vi "Select Level UI.vi"() -> (2 "Cancelled?":bool, 3 "Selected Level":string)   [LabVIEW 2020, in "App.lvlib" / "MazeUI.lvclass"]
uses:
  MazeUI.lvclass
  Maze/MazeGen/MazeGen.lvclass
panel:
  in  "Cancel":bool
  in  "Ok":bool
  in  "Level":i32(listbox)
  # "Select maze level:"
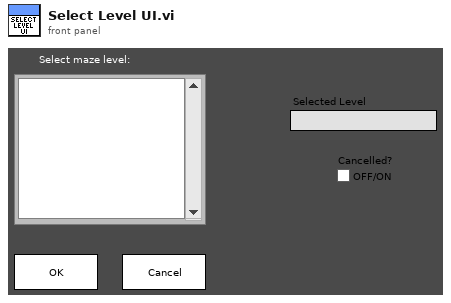
[diagram p1: front panel]
types:
  T1 = enum32{"Invalid", "Standard", "Closed", "Hidden", "Minimized", "Maximized"}
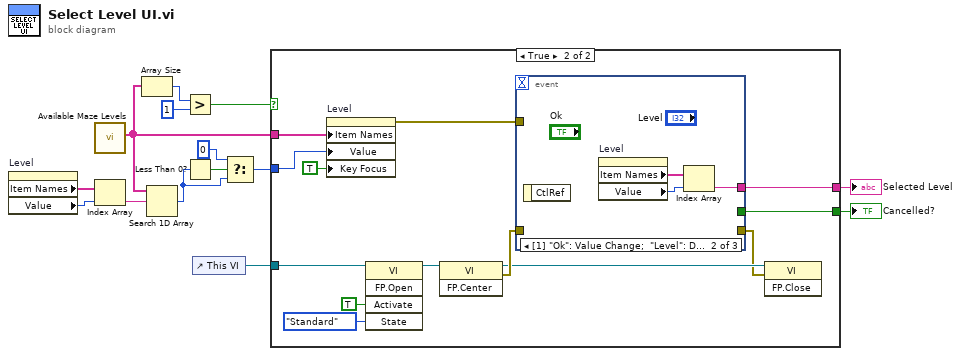
[diagram p0: block diagram]
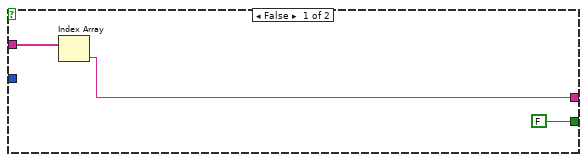
[diagram p2: hidden frame]
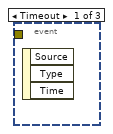
[diagram p3: hidden frame]
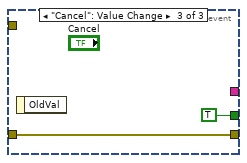
[diagram p4: hidden frame]
diagram:
  n1 = property on="Level" class="LstBox (strict)"() -> ("Item Names"=w14:string[], "Value"=w13:i32)  [unwired: 2 in, 2 out]
  n2 = call "Available Maze Levels.vi"() -> ("Names"=w3:string[])  [unwired: 10 in, 1 out]
  n3 = Index Array(array=w14, index=w13) -> (element=w2:string)
  n4 = Array Size(array=w3) -> (size(s)=w7:i32)
  n5 = Search 1D Array(1D array=w3, element=w2) -> (index of element=w1:i32)  [unwired: 1 in]
  n6 = Greater?(x=w7, y=1) -> (0:w5:bool)
  n7 = Less Than 0?(x=w1) -> (x < 0?=w12:bool)
  n8 = control-ref of="This VI"() -> (w4:refnum<vi>)
  n9 = Select(t=0, s=w12, f=w1) -> (s? t:f=w10:i32)
  n10 = case shown="True" w5 {
    tunnel: w10 -> [_ w30]
    tunnel: [w16 w27] -> w9
    tunnel: [FALSE w26] -> w8
    tunnel: w3 -> [w17 w25]
    tunnel: w4 -> [_ w24]
    frame False {
      n11 = Index Array(array=w17) -> (element=w16:string)  [unwired: 1 in]
    }
    frame True {
      n12 = property on="Level" class="LstBox (strict)"("Item Names"=w25, "Value"=w30, "Key Focus"=TRUE) -> (error out=w28:errorcluster)  [unwired: 2 in, 1 out]
      n13 = invoke class="VI" method="FP.Open"(reference=w24, "Activate"=TRUE ("Activate?"), "State"=T1."Standard") -> (reference out=w21:refnum<vi>)  [unwired: 2 in, 4 out]
      n14 = invoke class="VI" method="FP.Center"(reference=w21) -> (reference out=w19:refnum<vi>, error out=w20:errorcluster)  [unwired: 2 in, 1 out]
      n15 = event shown="[1] \"Ok\": Value Change;  \"Level\": Double Click" {
        selector: _ -> [_ _ _]
        dyn-events: _ -> [_ _ _]
        timeout: _ -> [_ _ _]
        tunnel: w28 -> [_ _ _]
        tunnel: [_ w31 _] -> w27
        tunnel: [_ _ TRUE] -> w26
        tunnel: w20 -> [_ _ w34]
        tunnel: [_ _ w34] -> w18
        event Timeout {
          n16 = event-data() -> ()  [unwired: 1 in, 3 out]
        }
        event "Ok": Value Change; "Level": Double Click {
          n17 = event-data() -> ()  [unwired: 1 in, 1 out]
          n18 = property on="Level" class="LstBox (strict)"() -> ("Item Names"=w33:string[], "Value"=w32:i32)  [unwired: 2 in, 2 out]
          n19 = Index Array(array=w33, index=w32) -> (element=w31:string)
        }
        event "Cancel": Value Change {
          n20 = event-data() -> ()  [unwired: 1 in, 1 out]
        }
      }
      n21 = invoke class="VI" method="FP.Close"(reference=w19, error in=w18) -> ()  [unwired: 1 in, 3 out]
    }
  }
  "Selected Level" <- w9
  "Cancelled?" <- w8
